vi "Bar Constructor.vi"(4 "Plot ID":i32, 8 "error in (no error)":errorcluster, 9 "z matrix":sgl[][](array[numeric]), 10 "y vector":sgl[](array[numeric]), 11 "3D Bar Datatype.lvclass in":refnum<class "3D Bar Datatype.lvclass">) -> (0 "error out":errorcluster, 3 "3D Bar Datatype.lvclass out":refnum<class "3D Bar Datatype.lvclass">)   [LabVIEW 2020, in "3D Bar Datatype.lvclass"]
uses:
  <vilib>/Math Plots/3D Math Plots/3D Bar/3D Bar Datatype/3D Bar Datatype.lvclass
  <vilib>/Math Plots/3D Math Plots/3D Bar/3D Bar Datatype/3D Bar Datatype.lvclass/3D Bar Datatype.ctl
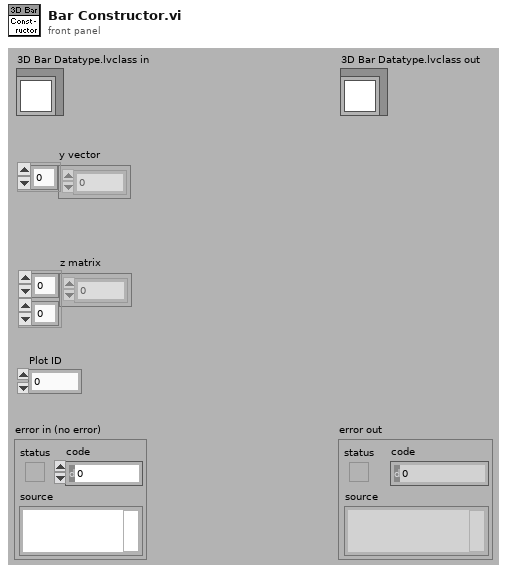
[diagram p1: front panel]
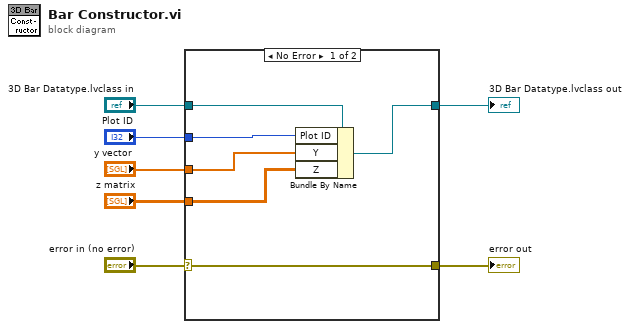
[diagram p0: block diagram]
diagram:
  n1 = case shown="No Error" "error in (no error)" {
    selector: "error in (no error)" -> [w9 w15]
    tunnel: "Plot ID" -> [w8 _]
    tunnel: [w9 w15] -> w6
    tunnel: "y vector" -> [w13 _]
    tunnel: "z matrix" -> [w12 _]
    tunnel: "3D Bar Datatype.lvclass in" -> [w11 w14]
    tunnel: [w10 w14] -> w1
    frame No Error {
      n2 = Bundle By Name(cluster=w11, "Plot ID"=w8, "Y"=w13, "Z"=w12) -> (w10:refnum<class "3D Bar Datatype.lvclass">)
    }
    frame Error {
    }
  }
  "error out" <- w6
  "3D Bar Datatype.lvclass out" <- w1
